vi "Add-action.vi"(8 "error in (no error)":errorcluster, 11 "Object ref in":T1) -> (0 "error out":errorcluster, 3 "Object ref out":T1)   [LabVIEW 2013, in "PowderDeposition.lvlib" / "PD-Main.lvclass"]
uses:
  PD-Main.lvclass
  Object-reference.ctl
  PD-Main.lvclass/PD-Main.ctl
  Assembly/Motor-assembly.lvclass
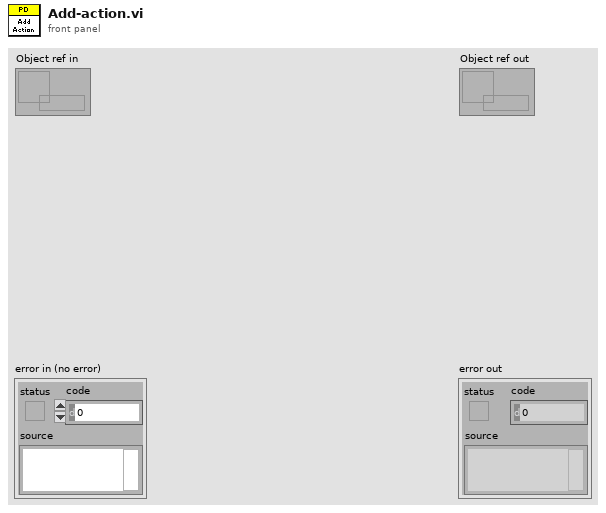
[diagram p1: front panel]
types:
  T1 = typedef "PowderDeposition.lvlib/PD-Main.lvclass/Object-reference.ctl" = refnum<data-value>
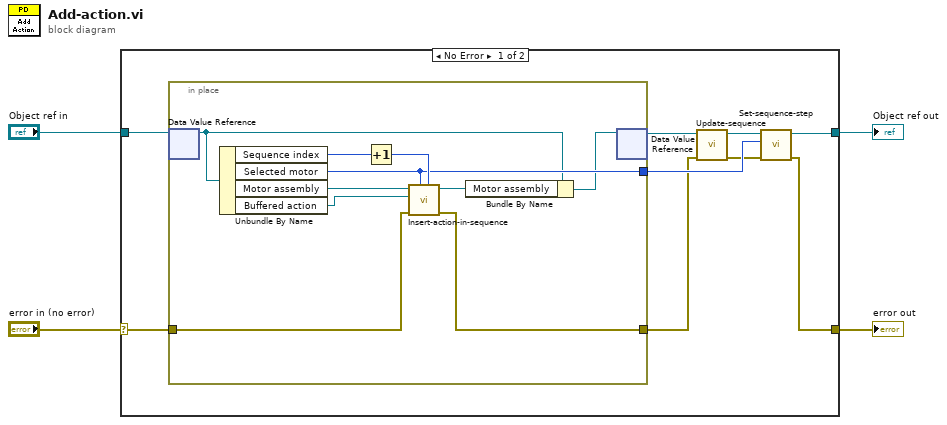
[diagram p0: block diagram]
diagram:
  n1 = case shown="No Error" "error in (no error)" {
    selector: "error in (no error)" -> [w13 w25]
    tunnel: [w10 w25] -> w3
    tunnel: [w12 w24] -> w1
    tunnel: "Object ref in" -> [w9 w24]
    frame No Error {
      n2 = in-place {
        in-place-border: w13 -> [w23]
        in-place-border: [w19] -> w11
        in-place-border: [w21] -> w6
        n3 = in-place-dvr #1(w9) -> (w16:refnum<class "PD-Main.lvclass">)  [unwired: 1 out]
        n4 = Unbundle By Name(w16) -> ("Sequence index"=w20:i32, "Selected motor"=w19:i32, "Motor assembly"=w18:refnum<class "Motor-assembly.lvclass">, "Buffered action"=w17:refnum<class "Action.lvclass">)
        n5 = Increment(x=w20) -> (x+1=w22:i32)
        n6 = call "Insert-action-in-sequence.vi"("Sequence index in"=w22, "Motor index"=w19, "error in (no error)"=w23, "Action"=w17, "Available motors in"=w18) -> ("error out"=w21:errorcluster, "Available motors out"=w15:refnum<class "Motor-assembly.lvclass">)  [unwired: 4 in, 1 out]
        n7 = Bundle By Name(cluster=w16, "Motor assembly"=w15) -> (w14:refnum<class "PD-Main.lvclass">)
        n8 = in-place-dvr #1(w14) -> (w8:T1)  [unwired: 1 out]
      }
      n9 = call "Update-sequence.vi"("error in (no error)"=w6, "Object ref in"=w8) -> ("error out"=w5:errorcluster, "Object ref out"=w7:T1)  [unwired: 8 in]
      n10 = call "Set-sequence-step.vi"("error in (no error)"=w5, "Sequence step in"=w11, "Object ref in"=w7) -> ("error out"=w10:errorcluster, "Object ref out"=w12:T1)  [unwired: 6 in, 1 out]
    }
    frame Error {
    }
  }
  "error out" <- w3
  "Object ref out" <- w1
